vi "SentinelDatalog.vi"(6 "error in":errorcluster, 8 "operation (0:open)":T1(ring)=enum."replace or create with confirmation", 10 "String":string, 11 "data log path":path) -> (0 "error out":errorcluster)   [LabVIEW 2011]
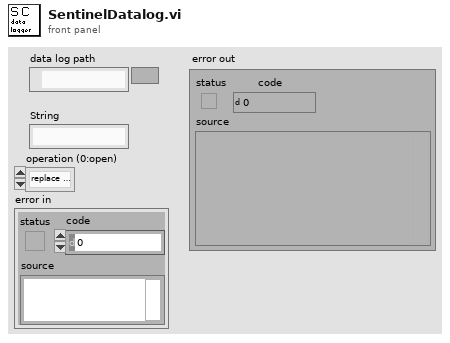
[diagram p1: front panel]
types:
  T1 = enum16{"open", "replace", "create", "open or create", "replace or create", "replace or create with confirmation"}
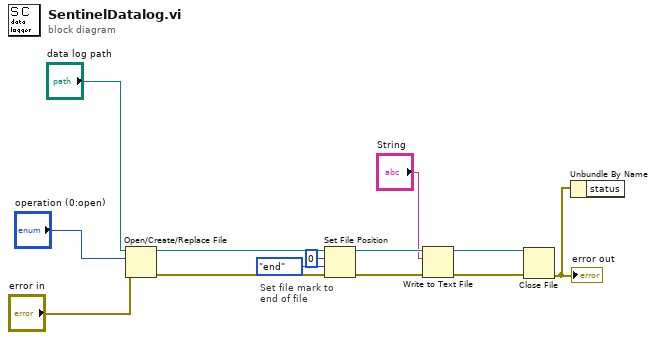
[diagram p0: block diagram]
diagram:
  # "Set file mark to\nend of file"
  n1 = Open/Create/Replace File(file path (use dialog)="data log path", error in="error in", operation (0:open)="operation (0:open)") -> (refnum out=w8:refnum<file>, error out=w7:errorcluster)  [unwired: 3 in, 1 out]
  n2 = Set File Position(offset (in bytes) (0)=i64 0, refnum=w8, from (0:start)=enum16{"start", "end", "current"}."end", error in=w7) -> (refnum out=w12:refnum<file>, error out=w13:errorcluster)
  n3 = Write to Text File(file (use dialog)=w12, text="String", error in=w13) -> (refnum out=w10:refnum<file>, error out=w11:errorcluster)  [unwired: 1 in, 1 out]
  n4 = Close File(refnum=w10, error in=w11) -> (error out=w2:errorcluster)  [unwired: 1 out]
  "error out" <- w2
  n5 = Unbundle By Name(w2) -> ()  [unwired: 1 out]
